vi "PI_GCS3_Configuration_Setup_SAM.vi"(0 "System no.":i32=1 min=1 step=1, 1 "Conn. Axes":string[](array[string]), 3 "Mode of Operation":T1[](array[typedef]), 5 "error in":errorcluster, 7 "Stop refnum":refnum<vi>) -> (19 "error out":errorcluster)   [LabVIEW 2026]
doc: "Select axis with specified drive state and waits until switched with SAM.\n\nRemark: Only referenced axes are allowed to change their drive state.\n\nWarning: Do not use this VI outside the GCS 3.0 Configuration Setup."
uses:
  SpecialCommand/ModeOfOperation.ctl
panel:
  # "Select axis with specified mode of operation and waits until switched with SAM.\n\nRemark: Only referenced axes are allowed\nto change their drive state.\n\nWarning: Do not use this VI outside the\nGCS 3.0 Configuration Setup."
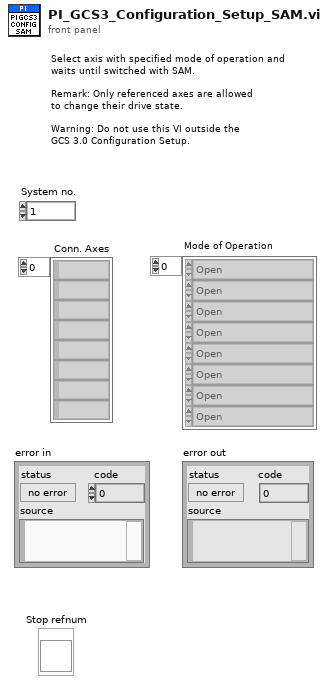
[diagram p1: front panel]
types:
  T1 = typedef "ModeOfOperation.ctl" = enum16{"Open", "Open-Loop Position", "Closed-Loop Position", "Open-Loop Velocity", "Closed-Loop Velocity", "Open-Loop Force", "Closed-Loop Force", "Step Operation"}
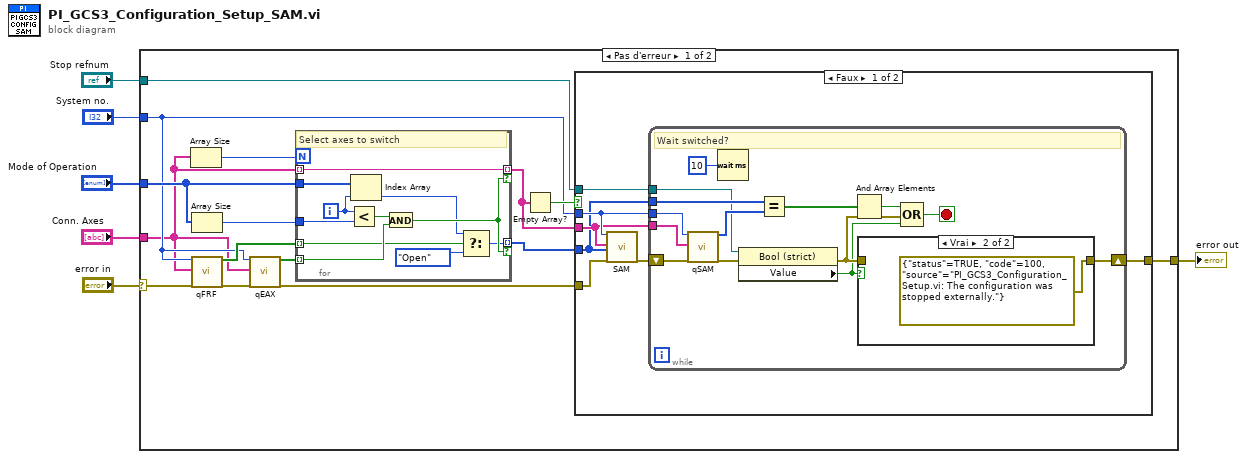
[diagram p0: block diagram]
diagram:
  n1 = case shown="Pas d'erreur" "error in" {
    selector: "error in" -> [w16 w57]
    tunnel: [w21 w57] -> w5
    tunnel: "Conn. Axes" -> [w7 _]
    tunnel: "Mode of Operation" -> [w17 _]
    tunnel: "System no." -> [w8 _]
    tunnel: "Stop refnum" -> [w19 _]
    frame No Error {
      n2 = Array Size(array=w7) -> (size(s)=w14:i32)
      n3 = Array Size(array=w17) -> (size(s)=w18:i32)
      n4 = call "qFRF.vi"("System no."=w8, "Axes to query"=w7, "error in"=w16) -> ("Referenced?"=w15:bool[], "error out"=w11:errorcluster)  [unwired: 15 in]
      n5 = call "qEAX.vi"("System no."=w8, "Axes to query"=w7, "error in"=w11) -> ("Axes enabled status"=w9:bool[], "error out"=w10:errorcluster)  [unwired: 15 in]
      n6 = for {
        N: w14 -> [_]
        tunnel: w17 -> [w31]
        tunnel: w18 -> [w32]
        tunnel: w15 -> [w22] mode=indexing
        tunnel: [w24] -> w13 mode=indexing if=w26
        tunnel: w7 -> [w29] mode=indexing
        tunnel: [w29] -> w12 mode=indexing if=w26
        tunnel: w9 -> [w27] mode=indexing
        i -> [w30]
        # "Select axes to switch"
        n7 = Less?(x=w30, y=w32) -> (x < y?=w28:bool)
        n8 = Index Array(array=w31, index=w30) -> (element=w23:T1)
        n9 = And(x=w28, y=w27) -> (x .and. y?=w26:bool)
        n10 = Select(t=w23, s=w22, f=ModeOfOperation."Open" ("y")) -> (s? t:f=w24:T1)
      }
      n11 = Empty Array?(array=w12) -> (empty?=w20:bool)
      n12 = case shown="Faux" w20 {
        tunnel: [w39 w56] -> w21
        tunnel: w10 -> [w37 w56]
        tunnel: w8 -> [w36 _]
        tunnel: w12 -> [w34 _]
        tunnel: w13 -> [w33 _]
        tunnel: w19 -> [w35 _]
        frame False {
          n13 = call "SAM.vi"("System no."=w36, "Axis"=w34, "Drive States"=w33, "error in"=w37) -> ("error out"=w38:errorcluster)  [unwired: 15 in]
          n14 = while {
            shift-right: [w44] -> w39
            shift-left: w38 -> [w53]
            tunnel: w36 -> [w52]
            tunnel: w34 -> [w51]
            tunnel: w33 -> [w49]
            tunnel: w35 -> [w45]
            stop <- w41 stop-if-true
            # "Wait switched?"
            n15 = call "qSAM.vi"("System no."=w52, "Axis"=w51, "error in"=w53) -> ("Mode of Operations"=w50:T1[], "error out"=w46:errorcluster)  [unwired: 15 in]
            n16 = Wait (ms)(milliseconds to wait=u32 10) -> ()  [unwired: 1 out]
            n17 = property class="Bool (strict)"(reference=w45, error in=w46) -> (error out=w42:errorcluster, "Value"=w40:bool)  [unwired: 1 out]
            n18 = Equal?(x=w49, y=w50) -> (x = y?=w48:bool[])
            n19 = And Array Elements(Boolean array=w48) -> (logical AND=w43:bool)
            n20 = case shown="Vrai" w40 {
              tunnel: [w54 errorcluster {"status"=TRUE, "code"=100, "source"="PI_GCS3_Configuration_Setup.vi: The configuration was stopped externally."} ("error out")] -> w44
              tunnel: w42 -> [w54 _]
              frame False {
              }
              frame True {
              }
            }
            n21 = Compound Arithmetic op=OR(w43, w42, w40) -> (w41:bool)
          }
        }
        frame True {
        }
      }
    }
    frame Error {
    }
  }
  "error out" <- w5
